vi "Decode_Int8.vi"(8 "error in (no error)":errorcluster, 10 "Registry Request":cluster{"Index":i32, "Length":i32}[](array[cluster]), 11 "navX Registry Cache in":refnum<class "navX Registry Cache.lvclass">) -> (0 "error out":errorcluster, 2 "Registry Response":i8[][](array[numeric]), 3 "navX Registry Cache out":refnum<class "navX Registry Cache.lvclass">)   [LabVIEW 2015, in "navX Library v3.lvlib" / "navX Registry Cache.lvclass"]
uses:
  navX Registry Cache.lvclass
  navX Registry Cache.lvclass/navX Registry Cache.ctl
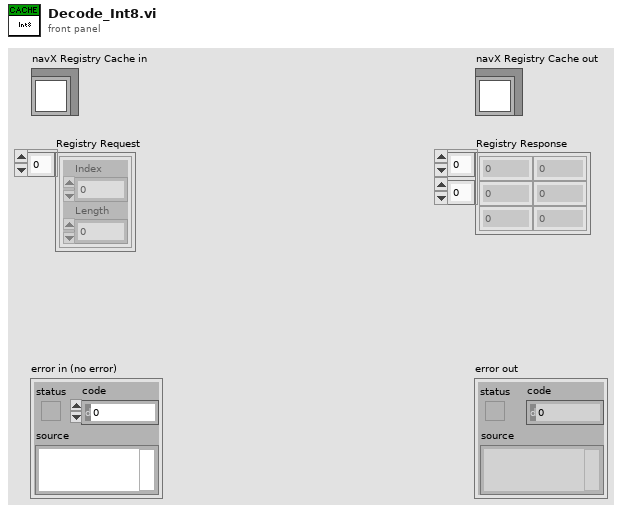
[diagram p1: front panel]
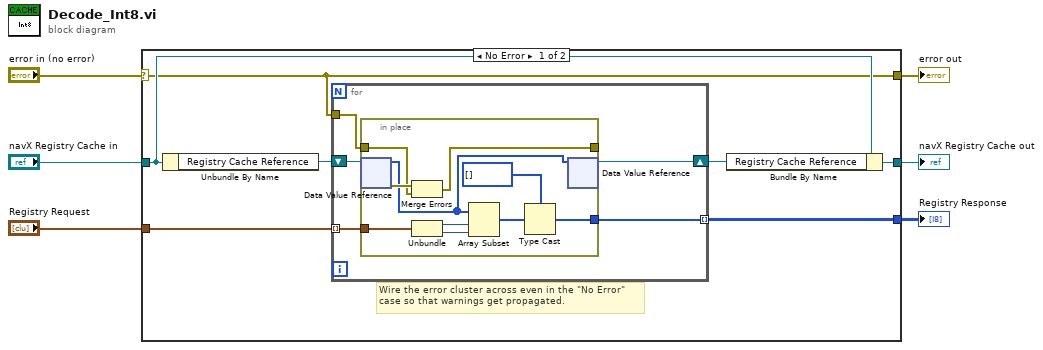
[diagram p0: block diagram]
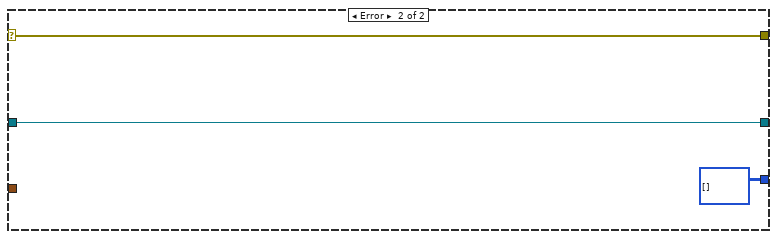
[diagram p2: hidden frame]
diagram:
  n1 = case shown="No Error" "error in (no error)" {
    selector: "error in (no error)" -> [w9 w31]
    tunnel: [w9 w31] -> w5
    tunnel: [w11 w30] -> w3
    tunnel: "navX Registry Cache in" -> [w12 w30]
    tunnel: "Registry Request" -> [w8 _]
    tunnel: [w7 i8[][] [] ("Int8")] -> w1
    frame No Error {
      # "Wire the error cluster across even in the \"No Error\"\ncase so that warnings get propagated."
      n2 = Unbundle By Name(w12) -> ("Registry Cache Reference"=w10:refnum<data-value>)
      n3 = for {
        tunnel: w9 -> [w16]
        tunnel: w8 -> [w15] mode=indexing
        shift-right: [w18] -> w13
        shift-left: w10 -> [w17]
        tunnel: [w14] -> w7 mode=indexing
        n4 = in-place {
          in-place-border: [w27] -> _
          in-place-border: w16 -> [w26]
          in-place-border: w15 -> [w24]
          in-place-border: [w19] -> w14
          n5 = in-place-dvr #1(w17) -> (w25:u8[], w28:errorcluster)
          n6 = Merge Errors(w28, w26) -> (w27:errorcluster)
          n7 = Unbundle(w24) -> ("Index"=w23:i32, "Length"=w22:i32)
          n8 = Array Subset(array=w25, index=w23, length=w22) -> (w20:u8[])
          n9 = Type Cast(type=i8[] [] ("Int8"), x=w20) -> (*(type *) &x=w19:i8[])
          n10 = in-place-dvr #1(w25) -> (w18:refnum<data-value>)  [unwired: 1 out]
        }
      }
      n11 = Bundle By Name(cluster=w12, "Registry Cache Reference"=w13) -> (w11:refnum<class "navX Registry Cache.lvclass">)
    }
    frame Error {
    }
  }
  "error out" <- w5
  "navX Registry Cache out" <- w3
  "Registry Response" <- w1
